vi "CONV String to 1D Boolean.vi"(0 "String":string, 1 "Delimiter (,)":string=",") -> (6 "1-D Boolean":bool[](array[boolean]))   [LabVIEW 2017]
doc: "This routine converts a string list to a 1-D Boolean array. \n\nThe Following Strings are treated as True (Non Case Sensitive):\n\n1\nT\nTrue\nOn\nYes\n\nAll other entries will be considered False.\n\nDelimiter input may be any character or characters. The entire Delimiter string will be treated as the delimiter. String input may or may not have a trailing delimiter.\n\nExample:\n\nString:\n1,F,On,False,No,True\n\nDelimiter:\n,\n\n1-D Boolean:\nT,F,T,F,F,T"
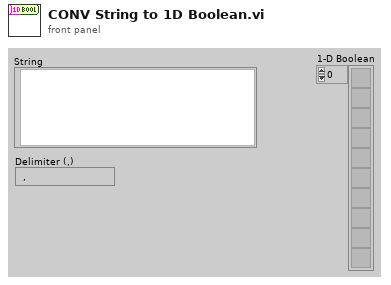
[diagram p1: front panel]
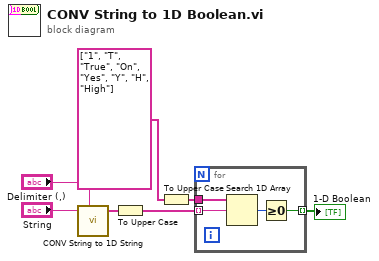
[diagram p0: block diagram]
diagram:
  n1 = call "CONV String to 1D String.vi"("String"="String", "Delimiter (,)"="Delimiter (,)") -> ("1-D String"=w2:string[])  [unwired: 7 out]
  n2 = To Upper Case(1:w2) -> (0:w1:string[])
  n3 = To Upper Case(1:string[] ["1", "T", "True", "On", "Yes", "Y", "H", "High"]) -> (0:w3:string[])
  n4 = for {
    tunnel: [w11] -> w5 mode=indexing
    tunnel: w3 -> [w9]
    tunnel: w1 -> [w8] mode=indexing
    n5 = Search 1D Array(1D array=w9, element=w8) -> (index of element=w10:i32)  [unwired: 1 in]
    n6 = Greater Or Equal To 0?(x=w10) -> (x >= 0?=w11:bool)
  }
  "1-D Boolean" <- w5
